vi "Calc.vi"(8 "error in (no error)":errorcluster, 11 "Y":dbl[](array[numeric])) -> (0 "error out":errorcluster, 1 "x-axis Shift":i32, 2 "properties":T1, 3 "graphs":dbl[][](array[numeric]))   [LabVIEW 2017, in "XGaussfitGraph.lvlib" / "XGaussfitGraph.xctl"]
doc: "Use this template to build a VI to use as a subVI."
uses:
  XGaussfitGraph.xctl
  Def-UI-Properties.ctl
  <vilib>/Analysis/6fits.llb/Curve Fitting Criteria.ctl
  <vilib>/Analysis/NI_AALPro.lvlib
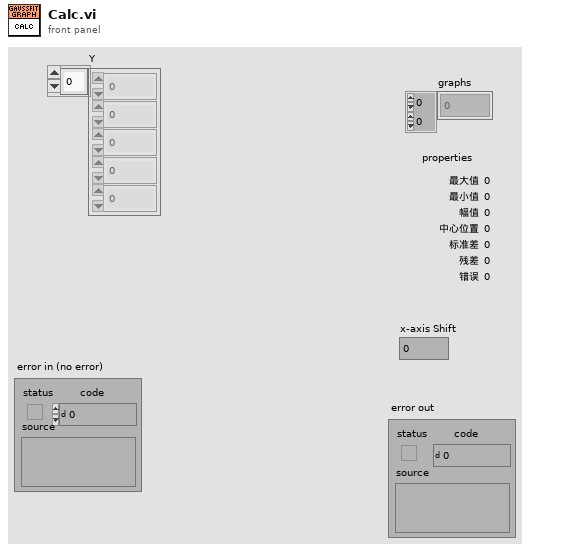
[diagram p1: front panel]
types:
  T1 = typedef "XGaussfitGraph.lvlib/XGaussfitGraph.xctl/Def-UI-Properties.ctl" = cluster{"max value":dbl, "min value":dbl, "amplitude":dbl, "center":dbl, "deviation":dbl, "residue":dbl, "error":i32}
  T2 = typedef "NI_AALPro.lvlib/Curve Fitting Criteria.ctl" = u16
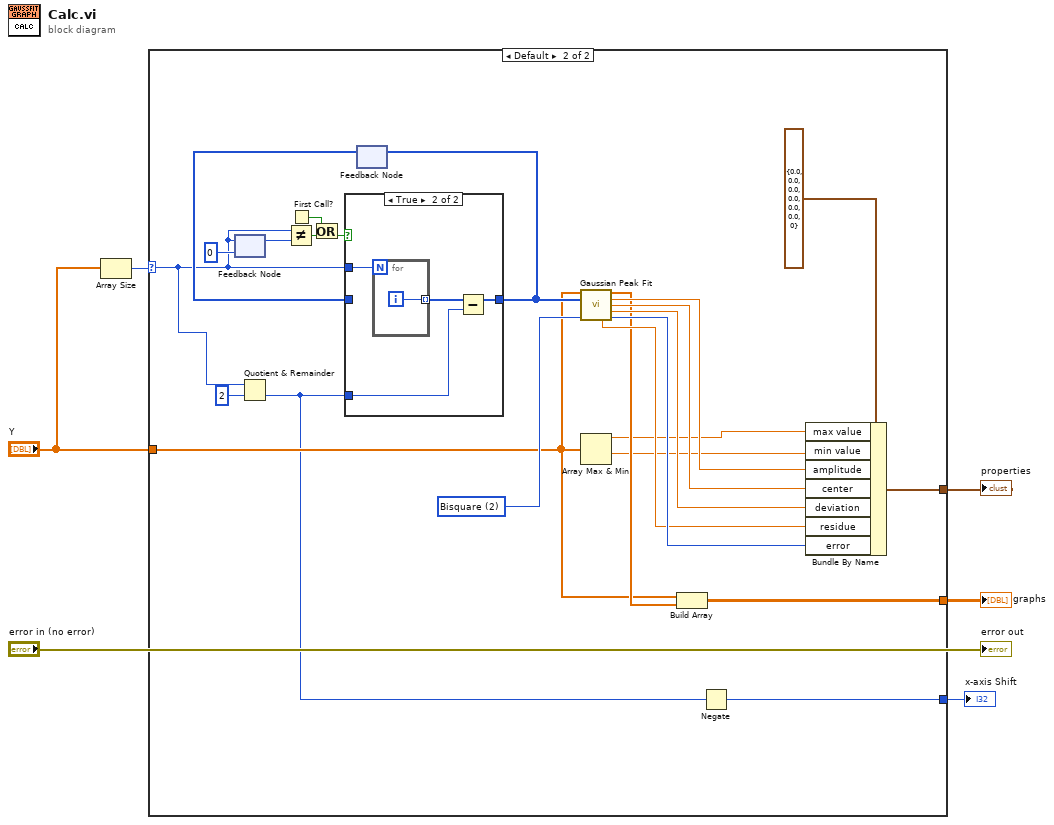
[diagram p0: block diagram]
diagram:
  n1 = Array Size(array="Y") -> (size(s)=w5:i32)
  n2 = case shown="Default" w5 {
    selector: w5 -> [_ w9]
    tunnel: "Y" -> [_ w16]
    tunnel: [_ w12] -> w3
    tunnel: [_ w11] -> w2
    tunnel: [_ w7] -> w1
    frame 0 {
    }
    frame Default {
      w17 = T2 2 items=["Least Square", "Least Absolute Residual", "Bisquare"] ("method")
      n3 = feedback #1(0) -> (w21:i32)
      n4 = feedback-in #1(w9) -> ()
      n5 = Quotient & Remainder(x=w9, y=2) -> (floor(x/y)=w8:i32)  [unwired: 1 out]
      n6 = Not Equal?(x=w9, y=w21) -> (x != y?=w22:bool)
      n7 = First Call?() -> (First Call?: T/F=w19:bool)
      n8 = Or(x=w19, y=w22) -> (x .or. y?=w20:bool)
      n9 = feedback #2() -> (w23:i32[])  [unwired: 1 in]
      n10 = case shown="True" w20 {
        tunnel: [w31 w34] -> w24
        tunnel: w9 -> [_ w33]
        tunnel: w23 -> [w31 _]
        tunnel: w8 -> [_ w32]
        frame False {
        }
        frame True {
          n11 = for {
            N: w33 -> [_]
            tunnel: [w36] -> w35 mode=indexing
            i -> [w36]
          }
          n12 = Subtract(x=w35, y=w32) -> (x-y=w34:i32[])
        }
      }
      n13 = feedback-in #2(w24) -> ()
      n14 = call <vilib>:"Gaussian Peak Fit.vi"("Y"=w16, "X"=w24, "method"=w17) -> ("Best Gaussian Fit"=w25:dbl[], "amplitude"=w30:dbl, "center"=w29:dbl, "standard deviation"=w28:dbl, "residue"=w26:dbl, "error"=w27:i32)  [unwired: 6 in, 1 out]
      n15 = Array Max & Min(array=w16) -> (max value=w15:dbl, min value=w14:dbl)  [unwired: 2 out]
      n16 = Build Array(w16, w25) -> (w11:dbl[][])
      n17 = Negate(x=w8) -> (-x=w7:i32)
      n18 = Bundle By Name(cluster=T1 {"max value"=0.0, "min value"=0.0, "amplitude"=0.0, "center"=0.0, "deviation"=0.0, "residue"=0.0, "error"=0} ("Charactor"), "max value"=w15, "min value"=w14, "amplitude"=w30, "center"=w29, "deviation"=w28, "residue"=w26, "error"=w27) -> (w12:T1)
    }
  }
  "properties" <- w3
  "graphs" <- w2
  "x-axis Shift" <- w1
  "error out" <- "error in (no error)"
